vi "Remove Command.vi"(8 "error in (no error)":errorcluster, 10 "Command Id":string, 11 "CommandDirector in":refnum<class "CommandDirector.lvclass">) -> (0 "error out":errorcluster, 1 "Removed?":bool, 2 "Removed Command":refnum<class "WriteCommand.lvclass">, 3 "CommandDirector out":refnum<class "CommandDirector.lvclass">)   [LabVIEW 2023, in "HAF.lvlib" / "CommandDirector.lvclass"]
doc: "Given an ID, finds and removes the Command from the collection that this Director holds. Returns an indication of whether or not the Command was found or not, and if it was the Command itself."
uses:
  CommandDirector.lvclass
  WriteCommand/WriteCommand.lvclass
  CommandDirector.lvclass/CommandDirector.ctl
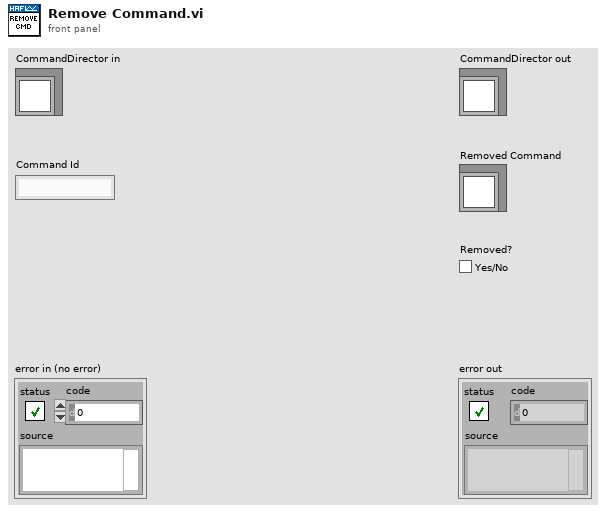
[diagram p1: front panel]
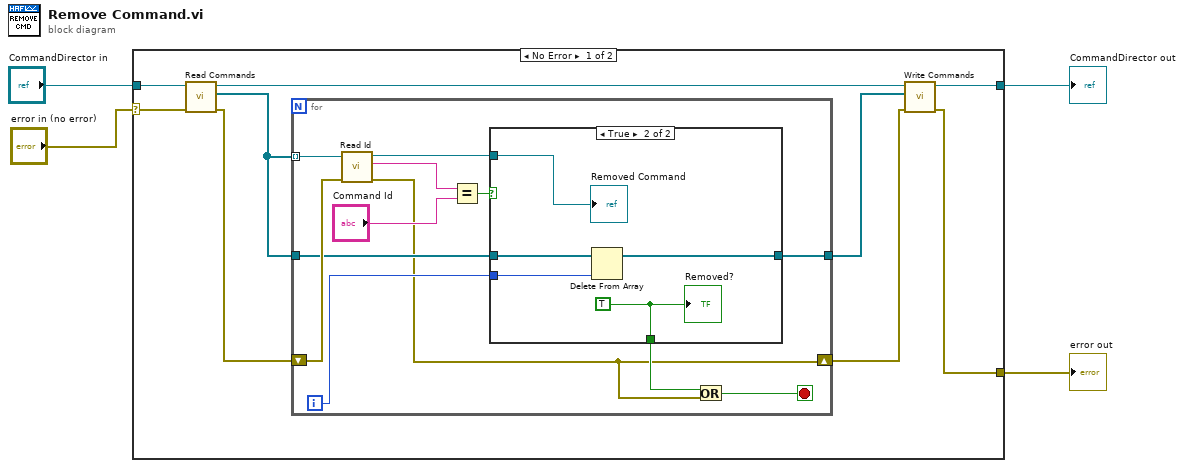
[diagram p0: block diagram]
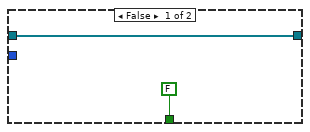
[diagram p2: hidden frame]
diagram:
  n1 = case shown="No Error" "error in (no error)" {
    selector: "error in (no error)" -> [w12 w34]
    tunnel: [w7 w34] -> w3
    tunnel: [w9 w33] -> w1
    tunnel: "CommandDirector in" -> [w13 w33]
    frame No Error {
      n2 = call-dynamic "Read Commands.vi"("error in (no error)"=w12, "CommandDirector in"=w13) -> ("error out"=w10:errorcluster, "Commands"=w11:refnum<class "WriteCommand.lvclass">[], "CommandDirector out"=w6:refnum<class "CommandDirector.lvclass">)  [unwired: 7 in]
      n3 = for {
        tunnel: w11 -> [w25] mode=indexing
        tunnel: w11 -> [w19]
        tunnel: [w17] -> w5
        shift-right: [w14] -> w8
        shift-left: w10 -> [w24]
        i -> [w18]
        stop <- w16 stop-if-true
        n4 = call-dynamic "Read Id.vi"("error in (no error)"=w24, "WriteCommand in"=w25) -> ("error out"=w14:errorcluster, "Id"=w23:string, "WriteCommand out"=w21:refnum<class "WriteCommand.lvclass">)  [unwired: 7 in]
        n5 = Equal?(x=w23, y="Command Id") -> (x = y?=w20:bool)
        n6 = case shown="True" w20 {
          tunnel: w21 -> [_ w32]
          tunnel: w19 -> [w27 w31]
          tunnel: w18 -> [_ w30]
          tunnel: [FALSE w29] -> w15
          tunnel: [w27 w28] -> w17
          frame False {
          }
          frame True {
            w29 = TRUE
            n7 = Delete From Array(array=w31, index=w30) -> (array with subset deleted=w28:refnum<class "WriteCommand.lvclass">[])  [unwired: 1 in, 1 out]
            "Removed Command" <- w32
            "Removed?" <- w29
          }
        }
        n8 = Or(x=w15, y=w14) -> (x .or. y?=w16:bool)
      }
      n9 = call-dynamic "Write Commands.vi"("error in (no error)"=w8, "Commands"=w5, "CommandDirector in"=w6) -> ("error out"=w7:errorcluster, "CommandDirector out"=w9:refnum<class "CommandDirector.lvclass">)  [unwired: 7 in]
    }
    frame Error {
    }
  }
  "error out" <- w3
  "CommandDirector out" <- w1
